vi "Convert LabVIEW Image Data To IMAQ.vi"(8 "error in (no error)":errorcluster, 10 "Image Data":T2, 11 "Image In":T1) -> (0 "error out":errorcluster, 3 "Image Out":T1)   [LabVIEW 2022 SP3]
doc: "This VI converts a LabVIEW Image into an IMAQ image."
uses:
  <vilib>/picture/picture.llb/imagedata.ctl
  <vilib>/vision/Image Controls.llb/IMAQ Image.ctl
  <vilib>/vision/NI_Vision_Development_Module.lvlib
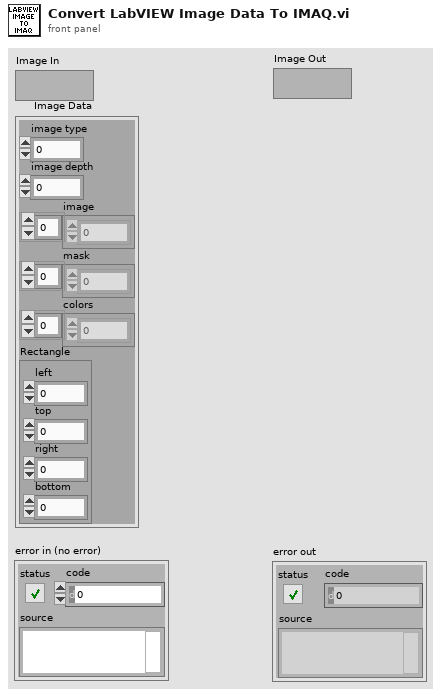
[diagram p1: front panel]
types:
  T1 = typedef "IMAQ Image.ctl" = refnum<image>
  T2 = typedef "imagedata.ctl" = cluster{"image type":i32, "image depth":i32, "image":u8[], "mask":u8[], "colors":u32[], "Rectangle":cluster{"left":i16, "top":i16, "right":i16, "bottom":i16}}
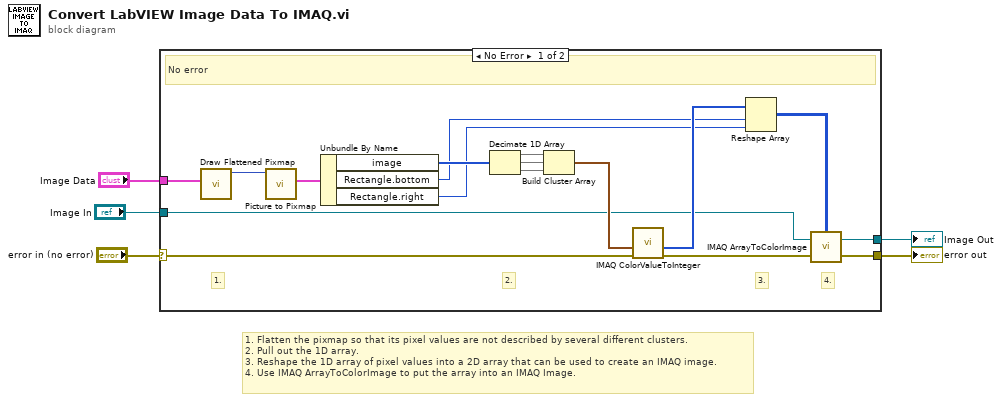
[diagram p0: block diagram]
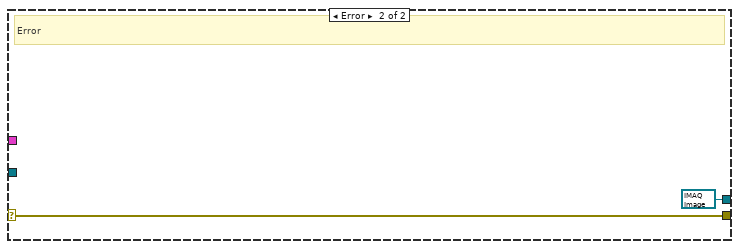
[diagram p2: hidden frame]
diagram:
  # "1. Flatten the pixmap so that its pixel values are not described by several different clusters.\n2. Pull out the 1D array.\n3. Reshape the 1D array of pixel values into a 2D array that can be used to create an IMAQ image.\n4. Use IMAQ ArrayToColorImage to put the array into an IMAQ Image."
  n1 = case shown="No Error" "error in (no error)" {
    selector: "error in (no error)" -> [w8 w24]
    tunnel: [w11 T1 refnum ("Image Out")] -> w5
    tunnel: [w9 w24] -> w4
    tunnel: "Image Data" -> [w7 _]
    tunnel: "Image In" -> [w6 _]
    frame No Error {
      # "4."
      # "3."
      # "2."
      # "1."
      # "No error"
      n2 = call <vilib>:"Draw Flattened Pixmap.vi"("image data"=w7) -> ("new picture"=w22:picture)  [unwired: 8 in]
      n3 = call <vilib>:"Picture to Pixmap.vi"("picture"=w22) -> ("image data"=w21:T2)  [unwired: 9 in, 1 out]
      n4 = Unbundle By Name(w21) -> ("image"=w20:u8[], "Rectangle.bottom"=w14:i16, "Rectangle.right"=w13:i16)
      n5 = Decimate 1D Array(w20) -> (w19:u8[], w18:u8[], w17:u8[])
      n6 = Build Cluster Array ("Index & Bundle Cluster Array")(w19, w18, w17) -> (w16:cluster{u8, u8, u8}[])
      n7 = call "IMAQ ColorValueToInteger"("error in (no error)"=w8, "1D Color value array"=w16) -> ("1D U32 array"=w15:u32[], "error out"=w10:errorcluster)  [unwired: 3 in, 2 out]
      n8 = Reshape Array(w15, w14, w13) -> (w12:u32[][])
      n9 = call "IMAQ ArrayToColorImage"("Image Pixels (U32)"=w12, "Image"=w6, "error in (no error)"=w10) -> ("Image Out"=w11:T1, "error out"=w9:errorcluster)  [unwired: 2 in]
    }
    frame Error {
      # "Error"
    }
  }
  "Image Out" <- w5
  "error out" <- w4
